vi "Convert Cursor Option to Cmd.vi"(7 "display option (on)":bool=TRUE, 11 "cursor option":T1(ring)=enum."cursor on & no blink") -> (3 "Display On Cmd":u8)   [LabVIEW 2017, in "HD44780 Common.lvlib"]
uses:
  HD44780 Common.lvlib
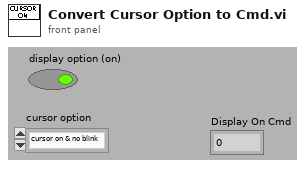
[diagram p1: front panel]
types:
  T1 = enum8{"cursor off", "cursor on & no blink", "cursor on & blink"}
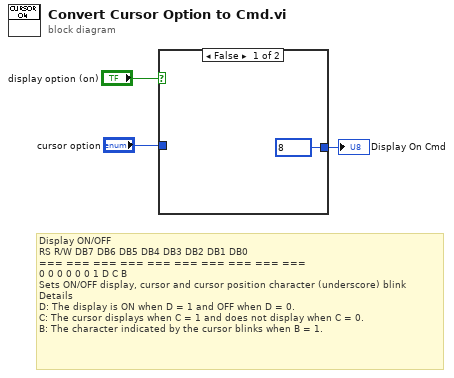
[diagram p0: block diagram]
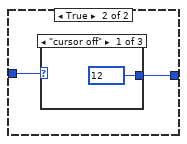
[diagram p2: hidden frame]
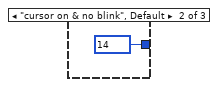
[diagram p3: hidden frame]
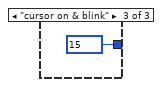
[diagram p4: hidden frame]
diagram:
  # "Display ON/OFF\nRS R/W DB7 DB6 DB5 DB4 DB3 DB2 DB1 DB0\n=== === === === === === === === === ===\n0 0 0 0 0 0 1 D C B\nSets ON/OFF display, cursor and cursor position character (underscore) blink\nDetails\nD: The display is ON when D = 1 and OFF when D = 0.\nC: The cursor displays when C = 1 and does not display when C = 0.\nB: The character indicated by the cursor blinks when B = 1."
  n1 = case shown="False" "display option (on)" {
    tunnel: [u8 8 ("LCD data/cmd") w6] -> w3
    tunnel: "cursor option" -> [_ w5]
    frame False {
    }
    frame True {
      n2 = case shown="\"cursor off\"" w5 {
        tunnel: [u8 12 ("LCD data/cmd") u8 14 ("LCD data/cmd") u8 15 ("LCD data/cmd")] -> w6
        frame "cursor off" {
        }
        frame "cursor on & no blink", Default {
        }
        frame "cursor on & blink" {
        }
      }
    }
  }
  "Display On Cmd" <- w3
